vi "Expand All.vi"(11 "Settings UI in":refnum<class "Settings UI.lvclass">) -> (3 "Settings UI out":refnum<class "Settings UI.lvclass">)   [LabVIEW 2020, in "Output Sequencer.lvlib" / "Settings UI.lvclass"]
uses:
  Settings UI.lvclass
  Settings UI.lvclass/Settings UI.ctl
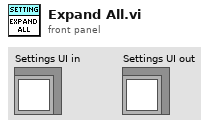
[diagram p1: front panel]
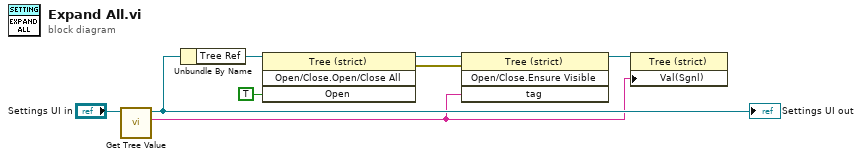
[diagram p0: block diagram]
diagram:
  n1 = call "Get Tree Value.vi"("UI Data in"="Settings UI in") -> ("Value"=w7:string, "UI Data out"=w8:refnum<class "Settings UI.lvclass">)  [unwired: 9 in]
  "Settings UI out" <- w8
  n2 = Unbundle By Name(w8) -> ("Tree Ref"=w2:refnum<vi>)
  n3 = invoke on="Invoke Node" class="Tree (strict)" method="Open/Close.Open/Close All"(reference=w2, "Open"=TRUE ("Open?")) -> (reference out=w4:refnum<vi>, error out=w5:errorcluster)  [unwired: 2 in, 2 out]
  n4 = invoke on="Invoke Node" class="Tree (strict)" method="Open/Close.Ensure Visible"(reference=w4, error in=w5, "tag"=w7) -> (reference out=w6:refnum<vi>)  [unwired: 1 in, 3 out]
  n5 = property class="Tree (strict)"(reference=w6, "Val(Sgnl)"=w7) -> ()  [unwired: 1 in, 2 out]
